vi "ROS_Topic_Write_Stop_Continuous_Primitive.vi"(3 "ROS in":T1={"topic port"=0, "Node"="", "topic"="", "type"="", "node port"=0, "error "={"status"=FALSE, "code"=0, "source"=""}, "Direction"=enum."Node", "Update (ms)"=1, "FIFO size"=1}) -> (1 "ROS out":T1={"topic port"=0, "Node"="", "topic"="", "type"="", "node port"=0, "error "={"status"=FALSE, "code"=0, "source"=""}, "Direction"=enum."Node", "Update (ms)"=1, "FIFO size"=1})   [LabVIEW 2015]
doc: "Instructs the server to stop publishing messages continuously."
uses:
  SubVIs/_ROSControl.ctl
  SubVIs/_ROSDirection.ctl
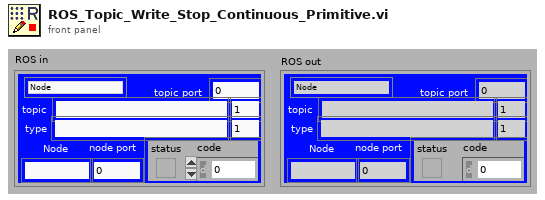
[diagram p1: front panel]
types:
  T1 = typedef "_ROSControl.ctl" = cluster{"topic port":u16, "Node":string, "topic":string, "type":string, "node port":u16, "error ":errorcluster, "Direction":T2, "Update (ms)":u16, "FIFO size":u16}
  T2 = typedef "_ROSDirection.ctl" = enum16{"Node", "Publisher", "Subscriber", "ServiceClient", "ServiceProvider"}
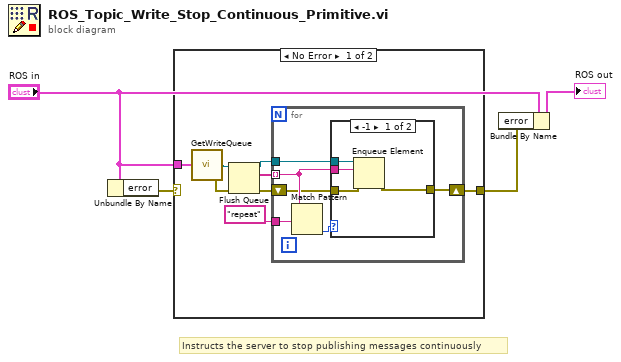
[diagram p0: block diagram]
diagram:
  # "Instructs the server to stop publishing messages continuously"
  n1 = Unbundle By Name("ROS in") -> ("error"=w1:errorcluster)
  n2 = case shown="No Error" w1 {
    selector: w1 -> [_ w24]
    tunnel: "ROS in" -> [w7 _]
    tunnel: [w8 w24] -> w2
    frame No Error {
      n3 = call "GetWriteQueue.vi"("ROS"=w7) -> ("error out"=w5:errorcluster, "queue out"=w6:refnum<queue>)  [unwired: 3 in]
      n4 = Flush Queue(queue=w6, error in (no error)=w5) -> (queue out=w9:refnum<queue>, remaining elements=w12:string[], error out=w10:errorcluster)
      n5 = for {
        tunnel: w12 -> [w16] mode=indexing
        tunnel: "repeat" ("regular expression") -> [w18]
        tunnel: w9 -> [w15]
        shift-right: [w13] -> w8
        shift-left: w10 -> [w14]
        n6 = Match Pattern(string=w16, regular expression=w18) -> (offset past match=w17:i32)  [unwired: 1 in, 3 out]
        n7 = case shown="-1" w17 {
          tunnel: w16 -> [w22 _]
          tunnel: w15 -> [w21 _]
          tunnel: [w20 w23] -> w13
          tunnel: w14 -> [w19 w23]
          frame -1 {
            n8 = Enqueue Element(queue=w21, element=w22, error in (no error)=w19) -> (error out=w20:errorcluster)  [unwired: 1 in, 2 out]
          }
          frame Default {
          }
        }
      }
    }
    frame Error {
    }
  }
  n9 = Bundle By Name(cluster="ROS in", "error"=w2) -> (→"ROS out":T1)
